vi "DI Callback 2 CPUs.vi"(11 "IRQ Number":u8) -> ()   [LabVIEW 2021]
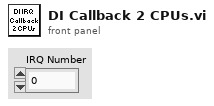
[diagram p1: front panel]
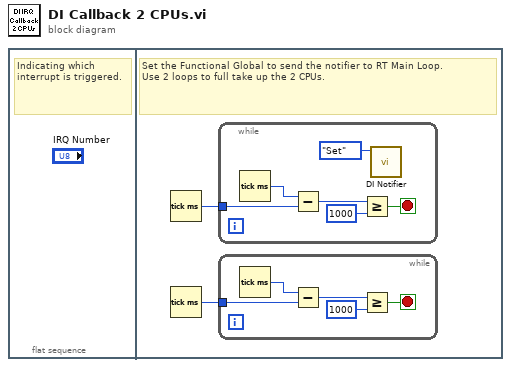
[diagram p0: block diagram]
diagram:
  n1 = flat-sequence {
    frame #0 {
      # "Indicating which interrupt is triggered."
    }
    frame #1 {
      # "Set the Functional Global to send the notifier to RT Main Loop. \nUse 2 loops to full take up the 2 CPUs."
      n2 = Tick Count (ms)() -> (millisecond timer value=w1:u32)
      n3 = Tick Count (ms)() -> (millisecond timer value=w2:u32)
      n4 = while {
        tunnel: w1 -> [w4]
        stop <- w5 stop-if-true
        n5 = Tick Count (ms)() -> (millisecond timer value=w6:u32)
        n6 = Subtract(x=w6, y=w4) -> (x-y=w7:u32)
        n7 = Greater Or Equal?(x=w7, y=u32 1000) -> (x >= y?=w5:bool)
        n8 = call "DI Notifier.vi"("Action"=enum16{"Get", "Set"}."Set") -> ()  [unwired: 10 in, 1 out]
      }
      n9 = while {
        tunnel: w2 -> [w9]
        stop <- w10 stop-if-true
        n10 = Tick Count (ms)() -> (millisecond timer value=w11:u32)
        n11 = Subtract(x=w11, y=w9) -> (x-y=w12:u32)
        n12 = Greater Or Equal?(x=w12, y=u32 1000) -> (x >= y?=w10:bool)
      }
    }
  }
